vi "worksheet write array formula num.vi"(0 "worksheet":u32, 1 "last_col":u16, 2 "format":u32, 5 "first_row":u32, 7 "first_col":u16, 9 "last_row":u32, 11 "error in (no error)":errorcluster, 12 "formula":string, 13 "result":dbl) -> (4 "function return":u32(ring), 15 "error out":errorcluster)   [LabVIEW 8.6]
doc: "lxw_error worksheet_write_array_formula_num(lxw_worksheet worksheet, lxw_row_t first_row, lxw_col_t first_col, lxw_row_t last_row, lxw_col_t last_col, const char *formula, lxw_format format, double result);"
uses:
  pending_lvxlsxwriter/xlsxwriter.dll
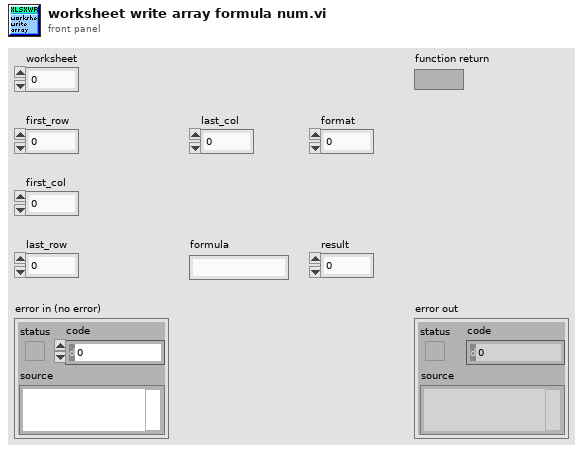
[diagram p1: front panel]
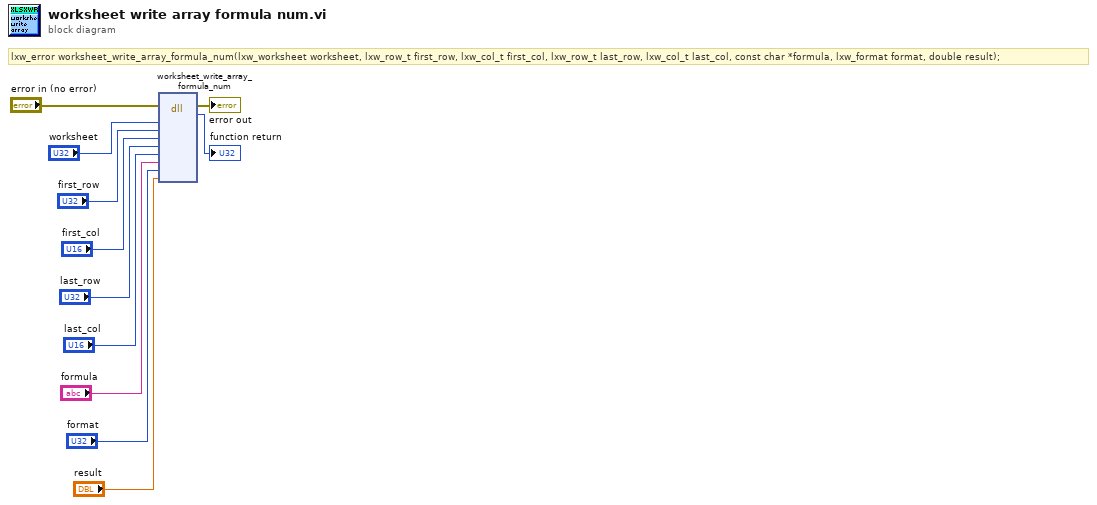
[diagram p0: block diagram]
diagram:
  # "lxw_error worksheet_write_array_formula_num(lxw_worksheet worksheet, lxw_row_t first_row, lxw_col_t first_col, lxw_row_t last_row, lxw_col_t last_col, const char *formula, lxw_format format, double result);"
  n1 = dll-call lib="C:/Users/WDAGUtilityAccount/Desktop/pending_lvxlsxwriter/xlsxwriter.*" fn="worksheet_write_array_formula_num"(error in="error in (no error)", "worksheet"="worksheet", "first_row"="first_row", "first_col"="first_col", "last_row"="last_row", "last_col"="last_col", "formula"="formula", "format"="format", "result"="result") -> (error out=→"error out":errorcluster, →"function return":u32)  [unwired: 10 in, 1 out]
